vi "Create HTTP Response (Status-Header-Body).vi"(5 "httpResponse":refnum<class "httpResponse.lvclass">, 8 "error in":errorcluster, 9 "body":string, 10 "Headers w/ status line(s)":string) -> (0 "error out":errorcluster, 3 "httpResponse out":refnum<class "httpResponse.lvclass">)   [LabVIEW 2020, in "httpClient.lvlib" / "httpResponse.lvclass"]
uses:
  httpResponse.lvclass
  httpResponse.lvclass/httpResponse.ctl
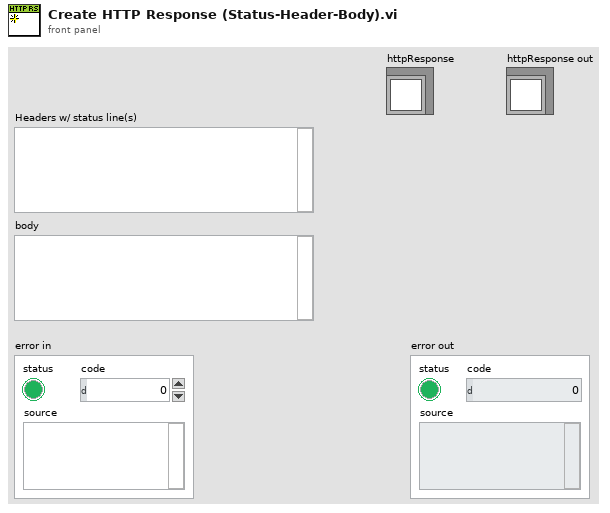
[diagram p1: front panel]
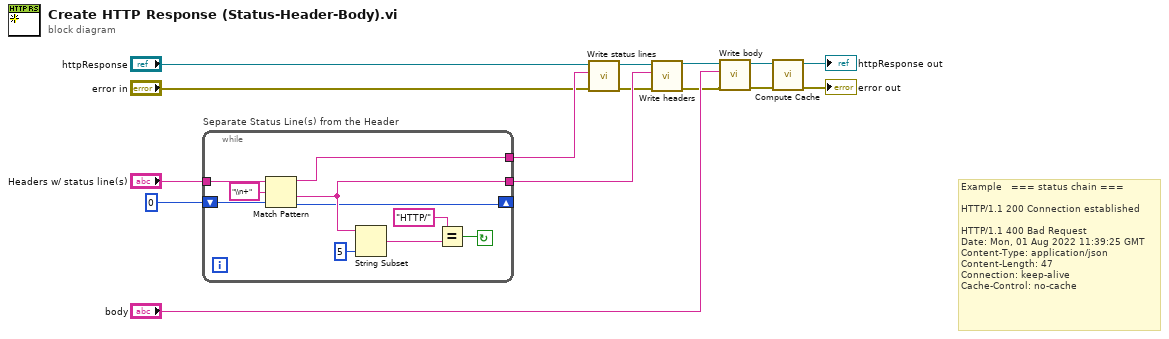
[diagram p0: block diagram]
diagram:
  # "Example   === status chain ===\n\nHTTP/1.1 200 Connection established\n\nHTTP/1.1 400 Bad Request\nDate: Mon, 01 Aug 2022 11:39:25 GMT\nContent-Type: application/json\nContent-Length: 47\nConnection: keep-alive\nCache-Control: no-cache"
  n1 = while "Separate Status Line(s) from the Header" {
    tunnel: [w24] -> w9
    shift-right: [w17] -> _
    shift-left: 0 ("offset (0)") -> [w18]
    tunnel: "Headers w/ status line(s)" -> [w25]
    tunnel: [w19] -> w10
    stop <- w20 continue-if-true
    n2 = Match Pattern(string=w25, regular expression="\\n+", offset (0)=w18) -> (before substring=w24:string, after substring=w19:string, offset past match=w17:i32)  [unwired: 1 out]
    n3 = String Subset(string=w19, length (rest)=5 ("length (rest)")) -> (substring=w21:string)  [unwired: 1 in]
    n4 = Equal?(x="HTTP/", y=w21) -> (x = y?=w20:bool)
  }
  n5 = call "Write status lines.vi"("error in (no error)"="error in", "status line"=w9, "httpResponse in"="httpResponse") -> ("error out"=w5:errorcluster, "httpResponse out"=w4:refnum<class "httpResponse.lvclass">)  [unwired: 7 in]
  n6 = call "Write headers.vi"("error in (no error)"=w5, "headers"=w10, "httpResponse in"=w4) -> ("error out"=w2:errorcluster, "httpResponse out"=w3:refnum<class "httpResponse.lvclass">)  [unwired: 7 in]
  n7 = call "Write body.vi"("error in (no error)"=w2, "body"="body", "httpRequest in"=w3) -> ("error out"=w11:errorcluster, "httpRequest out"=w12:refnum<class "httpResponse.lvclass">)  [unwired: 7 in]
  n8 = call "Compute Cache.vi"("error in (no error)"=w11, "httpResponse in"=w12) -> ("error out"=→"error out":errorcluster, "httpResponse out"=→"httpResponse out":refnum<class "httpResponse.lvclass">)  [unwired: 8 in]
